vi "sub_UnderBodyWash.vi"(8 "error in":errorcluster caption="에러 입력", 10 "Car Position Slider":refnum<vi>, 11 "Wash Options":refnum<vi>) -> (0 "error out":errorcluster caption="에러 출력", 2 "Elapsed Time (sec)":dbl format="%#.2g", 3 "Wash Indicators":T1)   [LabVIEW 2018]
uses:
  Control/Car Wash Indicators.ctl
  Control/Time.ctl
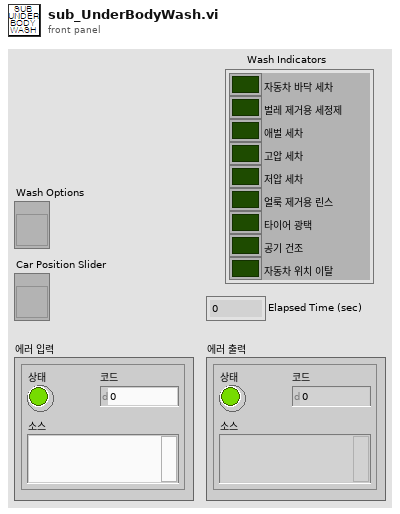
[diagram p1: front panel]
types:
  T1 = typedef "Car Wash Indicators.ctl" = cluster{"자동차 바닥 세차":bool, "벌레 제거용 세정제":bool, "애벌 세차":bool, "고압 세차":bool, "저압 세차":bool, "얼룩 제거용 린스":bool, "타이어 광택":bool, "공기 건조":bool, "자동차 위치 이탈":bool}
  T2 = enum8{"Enabled", "Disabled", "Disabled and Grayed Out"}
  T3 = typedef "Time.ctl" = enum16{"Start", "End"}
  T4 = typedef "Car Position Control.ctl" = i32
  T5 = typedef "Wash Options.ctl" = cluster{"Under Body Wash":bool, "Bug Remover":bool, "Pre-Soak":bool, "High Pressure Wash":bool, "Low Pressure Wax":bool, "Spot Free Rinse":bool, "Tire Shine Foam":bool, "Air Dry":bool}
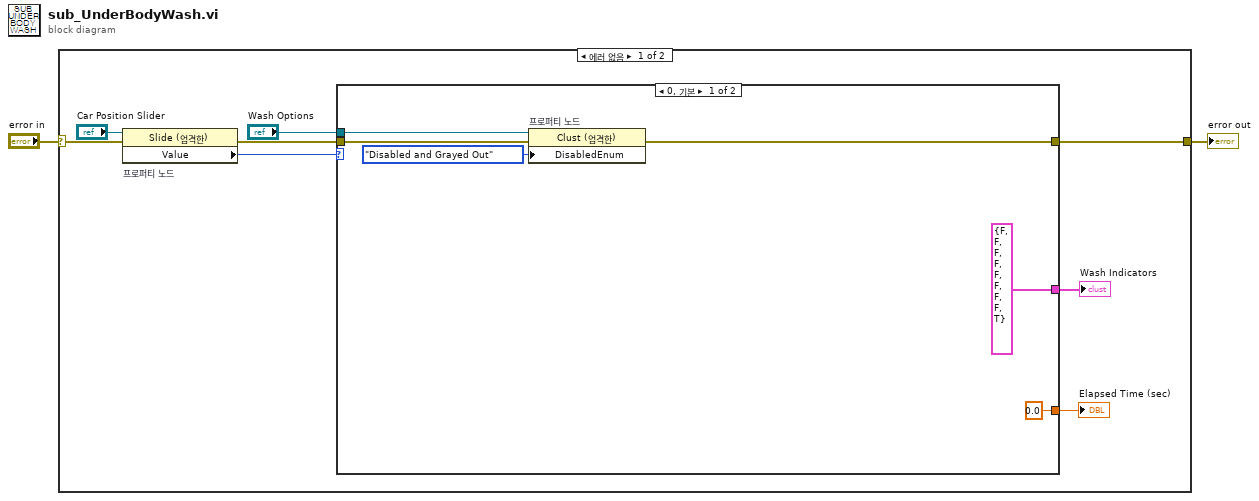
[diagram p0: block diagram]
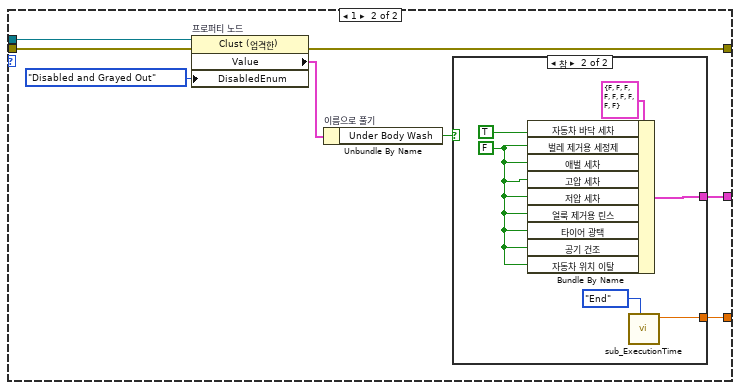
[diagram p2: hidden frame]
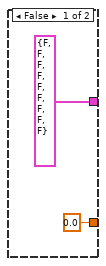
[diagram p3: hidden frame]
diagram:
  n1 = case shown="에러 없음" "error in" {
    selector: "error in" -> [w10 w33]
    tunnel: [w6 w33] -> w1
    frame No Error {
      n2 = property on="프로퍼티 노드" class="Slide (엄격한)"(reference="Car Position Slider", error in=w10) -> (error out=w8:errorcluster, "Value"=w7:T4)  [unwired: 1 out]
      n3 = case shown="0, 기본" w7 {
        tunnel: w8 -> [w14 w24]
        tunnel: [w11 w23] -> w6
        tunnel: [T1 {"자동차 바닥 세차"=FALSE, "벌레 제거용 세정제"=FALSE, "애벌 세차"=FALSE, "고압 세차"=FALSE, "저압 세차"=FALSE, "얼룩 제거용 린스"=FALSE, "타이어 광택"=FALSE, "공기 건조"=FALSE, "자동차 위치 이탈"=TRUE} ("Wash Indicators") w22] -> w5
        tunnel: [0.0 ("Elapsed Time (sec)") w19] -> w4
        tunnel: "Wash Options" -> [w13 w17]
        frame 0, Default {
          n4 = property on="프로퍼티 노드" class="Clust (엄격한)"(reference=w13, error in=w14, "DisabledEnum"=T2."Disabled and Grayed Out" ("비활성화")) -> (error out=w11:errorcluster)  [unwired: 1 out]
        }
        frame 1 {
          n5 = property on="프로퍼티 노드" class="Clust (엄격한)"(reference=w17, error in=w24, "DisabledEnum"=T2."Disabled and Grayed Out" ("비활성화")) -> (error out=w23:errorcluster, "Value"=w21:T5)  [unwired: 1 out]
          n6 = Unbundle By Name "이름으로 풀기"(w21) -> ("Under Body Wash"=w20:bool)
          n7 = case shown="참" w20 {
            tunnel: [T1 {"자동차 바닥 세차"=FALSE, "벌레 제거용 세정제"=FALSE, "애벌 세차"=FALSE, "고압 세차"=FALSE, "저압 세차"=FALSE, "얼룩 제거용 린스"=FALSE, "타이어 광택"=FALSE, "공기 건조"=FALSE, "자동차 위치 이탈"=FALSE} ("Wash Indicators") w31] -> w22
            tunnel: [0.0 ("Elapsed Time (sec)") w27] -> w19
            frame False {
            }
            frame True {
              w29 = FALSE ("Under Body Wash")
              n8 = Bundle By Name(cluster=T1 {"자동차 바닥 세차"=FALSE, "벌레 제거용 세정제"=FALSE, "애벌 세차"=FALSE, "고압 세차"=FALSE, "저압 세차"=FALSE, "얼룩 제거용 린스"=FALSE, "타이어 광택"=FALSE, "공기 건조"=FALSE, "자동차 위치 이탈"=FALSE} ("Wash Indicators"), "자동차 바닥 세차"=TRUE ("Under Body Wash"), "벌레 제거용 세정제"=w29, "애벌 세차"=w29, "고압 세차"=w29, "저압 세차"=w29, "얼룩 제거용 린스"=w29, "타이어 광택"=w29, "공기 건조"=w29, "자동차 위치 이탈"=w29) -> (w31:T1)
              n9 = call "sub_ExecutionTime.vi"("State"=Time."End") -> ("Elapsed Time (sec)"=w27:dbl)  [unwired: 9 in, 1 out]
            }
          }
        }
      }
      "Wash Indicators" <- w5
      "Elapsed Time (sec)" <- w4
    }
    frame Error {
    }
  }
  "error out" <- w1
